vi "FL_Filter_magnets_coordinates_(offline).vi"(7 "Data filtering":T1={"Filter type"=enum."Savitzky-Golay", "Length"=41, "Order"=3} {"Order" min=3 max=11 step=2; "Length" min=5 max=301 step=2}, 8 "error in (no error)":errorcluster, 11 "Magnets raw coordinates in":dbl[][](array[numeric])) -> (0 "error out":errorcluster, 3 "Magnets filtered coordinates out":dbl[][](array[numeric]))   [LabVIEW 2018, in "Tracker.lvlib"]
uses:
  Tracker.lvlib
  Controls/CTL_Filter_selector.ctl
  <vilib>/Analysis/3filter.llb/Savitzky-Golay Filter (DBL).vi
  <vilib>/Analysis/NI_AALBase.lvlib
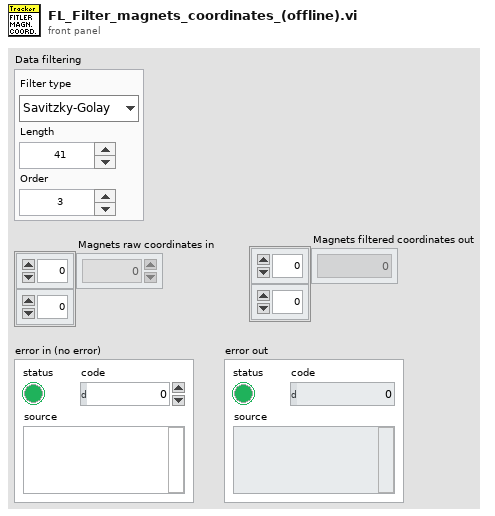
[diagram p1: front panel]
types:
  T1 = typedef "Tracker.lvlib/CTL_Filter_selector.ctl" = cluster{"Filter type":enum16{"None", "Savitzky-Golay"}, "Length":i32, "Order":i32}
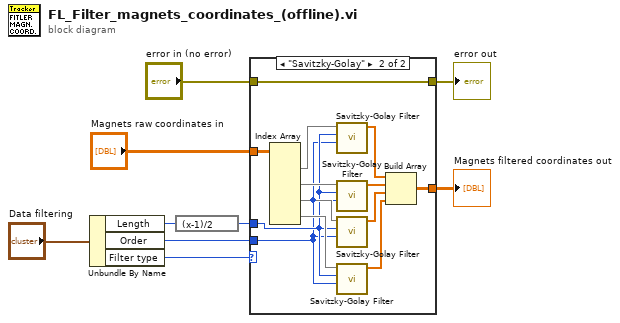
[diagram p0: block diagram]
diagram:
  n1 = Unbundle By Name("Data filtering") -> ("Length"=w4:i32, "Order"=w6:i32, "Filter type"=w7:enum16{"None", "Savitzky-Golay"})
  n2 = expression code="(x-1)/2"(w4) -> (w5:i32)
  n3 = case shown="\"Savitzky-Golay\"" w7 {
    tunnel: "Magnets raw coordinates in" -> [w11 w24]
    tunnel: w5 -> [_ w19]
    tunnel: w6 -> [_ w18]
    tunnel: [w11 w13] -> w1
    tunnel: [w10 w12] -> w8
    tunnel: "error in (no error)" -> [w10 w12]
    frame "None", Default {
    }
    frame "Savitzky-Golay" {
      n4 = Index Array(array=w24) -> (element #1=w23:dbl[], element #2=w22:dbl[], element #3=w21:dbl[], element #4=w20:dbl[])  [unwired: 8 in]
      n5 = call-poly <vilib>:"Savitzky-Golay Filter.vi"("polynomial order"=w18, "side points"=w19, "X"=w23) -> ("Filtered X"=w17:dbl[])  [unwired: 7 in, 1 out]
      n6 = call-poly <vilib>:"Savitzky-Golay Filter.vi"("polynomial order"=w18, "side points"=w19, "X"=w22) -> ("Filtered X"=w16:dbl[])  [unwired: 7 in, 1 out]
      n7 = call-poly <vilib>:"Savitzky-Golay Filter.vi"("polynomial order"=w18, "side points"=w19, "X"=w21) -> ("Filtered X"=w15:dbl[])  [unwired: 7 in, 1 out]
      n8 = call-poly <vilib>:"Savitzky-Golay Filter.vi"("polynomial order"=w18, "side points"=w19, "X"=w20) -> ("Filtered X"=w14:dbl[])  [unwired: 7 in, 1 out]
      n9 = Build Array(w17, w16, w15, w14) -> (w13:dbl[][])
    }
  }
  "error out" <- w8
  "Magnets filtered coordinates out" <- w1
